vi "cnvrt_nmVac_waveNr.vi"(0 "wavelength (nm vac)":dbl format="%.2f", 5 "error in (no error)":errorcluster) -> (14 "waveNr":dbl format="%.2f", 19 "error out":errorcluster)   [LabVIEW 2010, in "OSA.lvclass"]
uses:
  OSA.lvclass
  FTSLib.dll
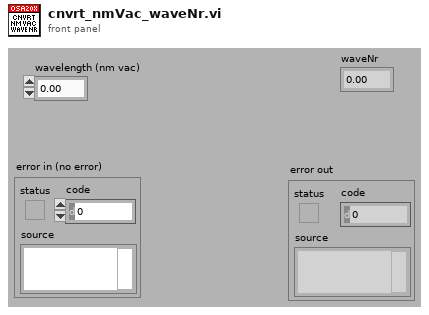
[diagram p1: front panel]
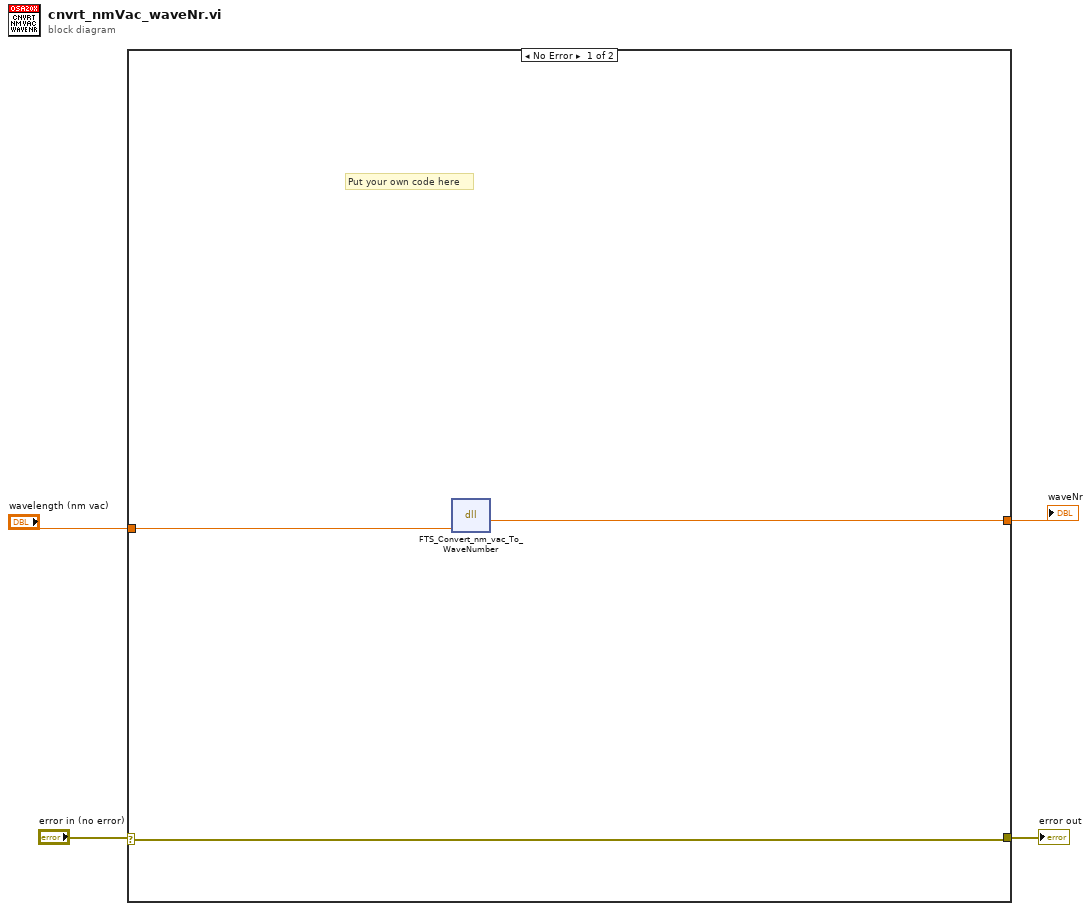
[diagram p0: block diagram]
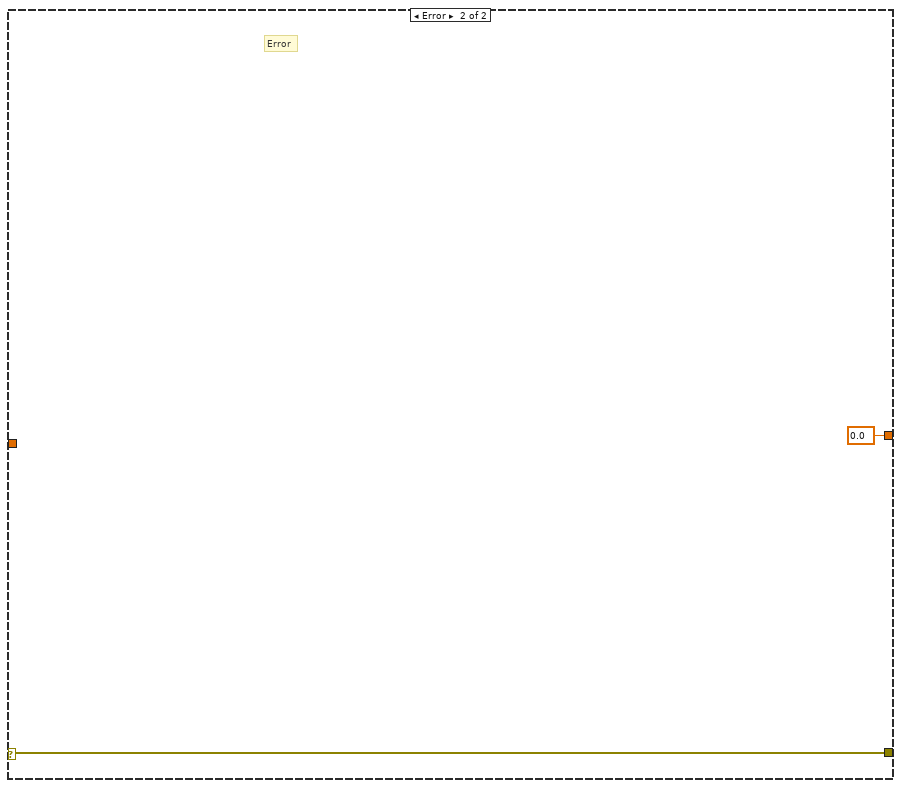
[diagram p2: hidden frame]
diagram:
  n1 = case shown="No Error" "error in (no error)" {
    selector: "error in (no error)" -> [w5 w9]
    tunnel: [w5 w9] -> w4
    tunnel: "wavelength (nm vac)" -> [w7 _]
    tunnel: [w6 0.0] -> w1
    frame No Error {
      # "Put your own code here"
      n2 = dll-call lib="FTSLib.dll" fn="FTS_Convert_nm_vac_To_WaveNumber"("wavelength"=w7) -> ("return type"=w6:dbl)  [unwired: 4 in, 2 out]
    }
    frame Error {
      # "Error"
    }
  }
  "error out" <- w4
  "waveNr" <- w1
